vi "NATS JetStream Server Start w Config Windows.vi"(6 "Timeout (1000 ms)":i32=1000, 7 "NATS Server EXE Path (default install)":path, 8 "error in":errorcluster, 11 "Config File":path) -> (0 "error out":errorcluster, 3 "Active?":bool)   [LabVIEW 2020, in "NATS Infrastructure.lvlib"]
doc: "Stops NATS server on Windows machines."
uses:
  NATS Infrastructure.lvlib
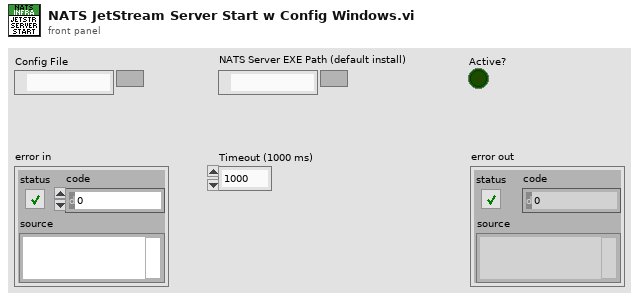
[diagram p1: front panel]
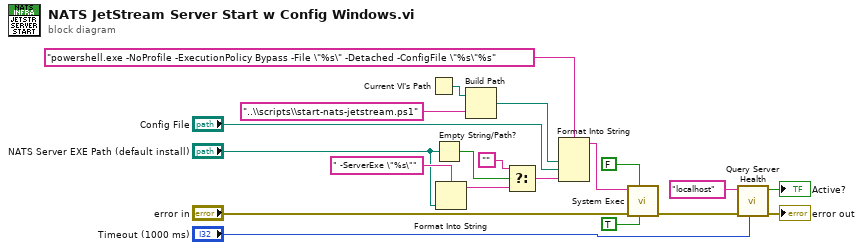
[diagram p0: block diagram]
diagram:
  n1 = Current VI's Path() -> (path=w14:path)
  n2 = Empty String/Path?(string/path="NATS Server EXE Path (default install)") -> (empty?=w10:bool)
  n3 = Format Into String(format string=" -ServerExe \"%s\"", "NATS Server EXE Path (default install)") -> (resulting string=w9:string)  [unwired: 2 in, 1 out]
  n4 = Build Path(base path=w14, name or relative path="..\\scripts\\start-nats-jetstream.ps1") -> (appended path=w13:path)
  n5 = Select(t="", s=w10, f=w9) -> (s? t:f=w6:string)
  n6 = Format Into String(format string="powershell.exe -NoProfile -ExecutionPolicy Bypass -File \"%s\" -Detached -ConfigFile \"%s\"%s" ("command line"), w13, "Config File", w6) -> (resulting string=w16:string)  [unwired: 2 in, 1 out]
  n7 = call <vilib>:"System Exec.vi"("run minimized? (F)"=TRUE ("run minimized (T)"), "wait until completion? (T)"=FALSE, "error in (no error)"="error in", "command line"=w16) -> ("error out"=w5:errorcluster)  [unwired: 4 in, 3 out]
  n8 = call "Query Server Health.vi"("Timeout (1000 ms)"="Timeout (1000 ms)", "error in"=w5, "Server Address (localhost)"="localhost") -> ("error out"=→"error out":errorcluster, "healthy"=→"Active?":bool)  [unwired: 7 in]
